vi "init UI.vi"(5 "Sub Panel":refnum<vi>, 6 "node ref":T9, 8 "Top VI":refnum<vi>, 9 "Enum in":refnum<vi>, 10 "Listbox":refnum<vi>, 11 "References in":T2) -> (0 "error out":errorcluster, 1 "Objects out":T1, 2 "Event Registration Refnum":refnum<event-registration>, 3 "References out":T2, 4 "Multi Column Listbox out":refnum<class "Multi Column Listbox.lvclass">)   [LabVIEW 2013, in "Scaling editor node.lvclass"]
uses:
  Scaling editor node.lvclass
  <vilib>/NI/Configuration Framework/Node/NodeRef.ctl
  <vilib>/NI/Configuration Framework/Node/NISE_CEF_Node.lvclass
  <vilib>/NI/DCAF Table API/Table Manager/references.ctl
  <vilib>/NI/Configuration Framework/Node/StopEvent.ctl
  <vilib>/NI/Configuration Framework/Node/RefreshUIEvent.ctl
  <vilib>/NI/Configuration Framework/Node/CacheState.ctl
  <vilib>/NI/Configuration Framework/Node/NodeChangeEvent.ctl
  <vilib>/NI/Tag Bus Data Framework/control module/editor node/channel action event.ctl
  <vilib>/NI/Tag Bus Data Framework/control module/editor node/dialog output action.ctl
  <vilib>/NI/Tag Bus Module Framework/channel/TBM channel.lvclass
  <vilib>/NI/Tag Bus/tag/tag descriptor.lvclass
  <vilib>/NI/AMC/Message Queue.ctl
  <vilib>/NI/AMC/Message.ctl
  <vilib>/NI/Tools/Keyed Array/KeyedArray.ctl
  <vilib>/NI/Configuration Framework/Node/UserEventRef.ctl
  <vilib>/NI/Configuration Framework/Controls/EventCluster.ctl
  <vilib>/NI/DCAF Table API/Table Manager/object ref.ctl
  <vilib>/NI/Tag Bus Data Framework/Configuration Editor/Classes/Engine Parent/Engine Parent Editor Node.lvclass
  <vilib>/NI/Tag Bus Data Framework/Configuration Editor/Classes/Module editor node/module editor node.lvclass
  <vilib>/NI/DCAF Table API/Listbox/Multi Column Listbox.lvclass
  <vilib>/NI/DCAF Table API/Listbox/Multi Column Listbox.lvclass/Multi Column Listbox.ctl
  <vilib>/NI/DCAF Table API/Table Manager/Table Manager.lvclass/Table Manager.ctl
  <vilib>/NI/DCAF Table API/Listbox/Write Listbox.vi
  <vilib>/NI/DCAF Table API/Table Manager/Write Top VI.vi
  <vilib>/NI/DCAF Table API/Table Manager/Table Manager.lvclass
  <vilib>/NI/Tag Bus Data Framework/control module/editor node/control module editor.lvclass
  <vilib>/NI/Tools/Keyed Array/Tools_KeyedArray.lvlib
  <vilib>/NI/AMC/AMC.lvlib
  <vilib>/NI/Configuration Framework/NISE_CEF_TreeControl.lvlib
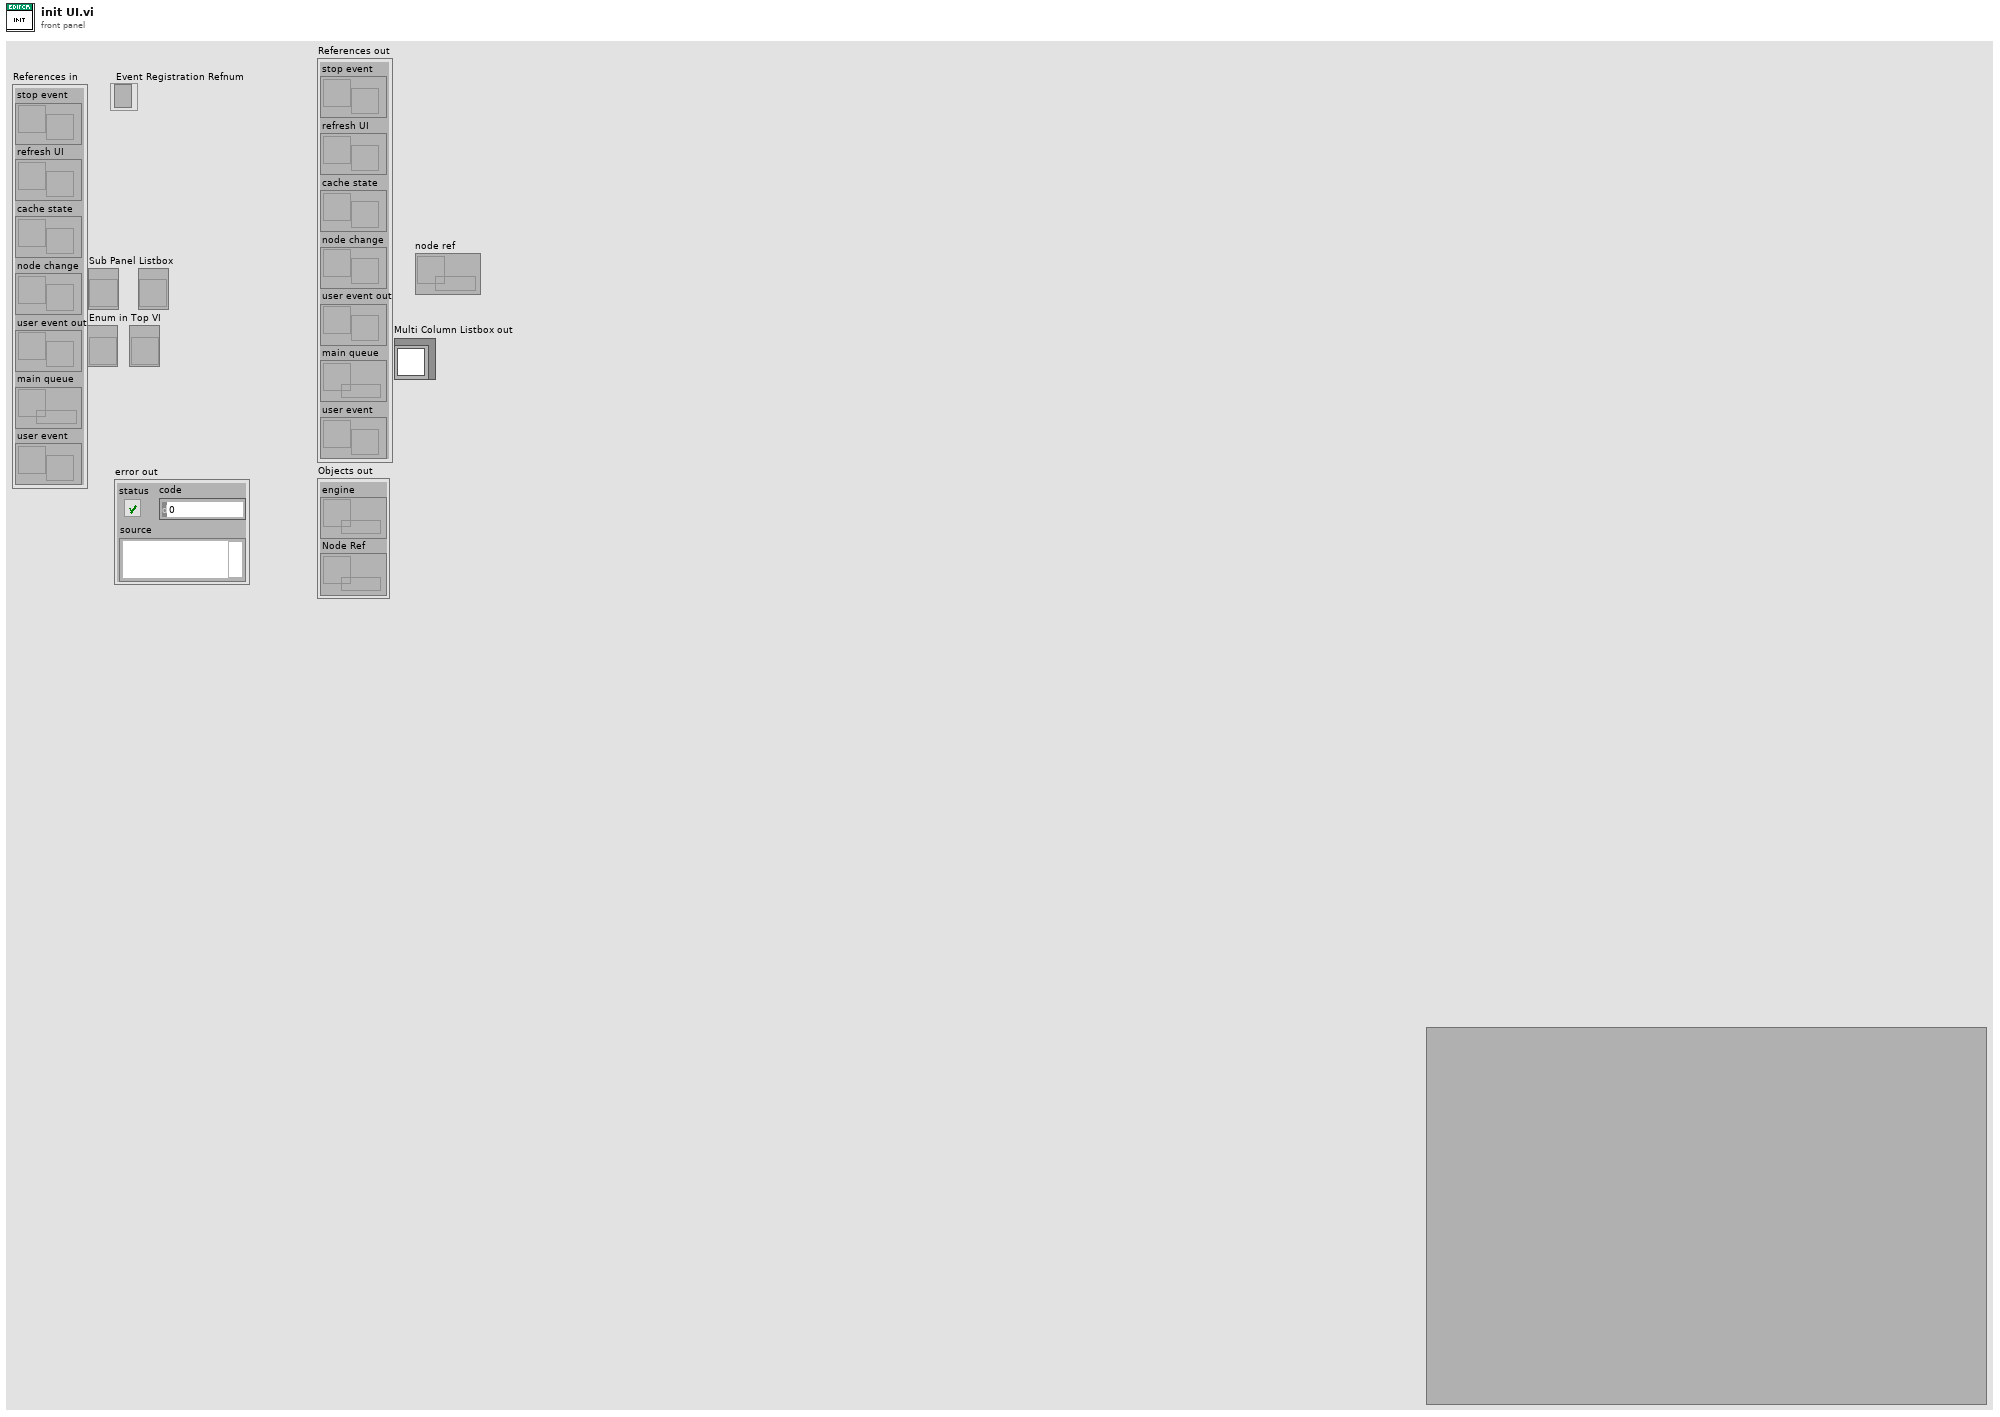
[diagram p1: front panel]
types:
  T1 = typedef "Table Manager.lvlib/Table Manager.lvclass/object ref.ctl" = cluster{"engine":refnum<data-value>, "Node Ref":refnum<data-value>}
  T2 = typedef "Table Manager.lvlib/Table Manager.lvclass/references.ctl" = cluster{"stop event":T3, "refresh UI":T4, "cache state":T5, "node change":T6, "user event out":refnum<user-event>, "main queue":T7, "user event":T8}
  T3 = typedef "NISE_CEF_Node.lvclass/StopEvent.ctl" = refnum<user-event>
  T4 = typedef "NISE_CEF_Node.lvclass/RefreshUIEvent.ctl" = refnum<user-event>
  T5 = typedef "NISE_CEF_Node.lvclass/CacheState.ctl" = refnum<user-event>
  T6 = typedef "NISE_CEF_Node.lvclass/NodeChangeEvent.ctl" = refnum<user-event>
  T7 = typedef "AMC.lvlib/Message Queue.ctl" = refnum<queue>
  T8 = typedef "NISE_CEF_Node.lvclass/UserEventRef.ctl" = refnum<user-event>
  T9 = typedef "NISE_CEF_Node.lvclass/NodeRef.ctl" = refnum<data-value>
  T10 = typedef "Table Manager.lvlib/Column.lvclass/Column Descriptor.ctl" = cluster{"name":string, "caption":string, "Column Type":T11, "Params":string, "AutoSizeMode":i32, "FillWeight":sgl, "MinWidth":u32, "tooltip":string, "Enum Reference":refnum<vi>, "Channel suffix":string, "Read Only":bool, "Call Back VI":T12, "DT Dependency":i32, "name dependency":i32, "data type":T13}
  T11 = typedef "Table Manager.lvlib/Column.lvclass/Column Type.ctl" = enum16{"String", "Mapping", "Channel Name", "Tag", "Enum", "Data Type", "Numeric"}
  T12 = typedef "Table Manager.lvlib/Table Manager.lvclass/Call Back Ref Type Def.ctl" = refnum<vi>
  T13 = typedef "tag bus.lvlib/tag descriptor.lvclass/Data Type.ctl" = enum16{"Double", "Single", "I64", "I32", "I16", "I8", "U64", "U32", "U16", "U8", "Boolean", "String", "Array of Double", "Array of Single", "Array of I64", "Array of I32", "Array of I16", "Array of I8", "Array of U64", "Array of U32", "Array of U16", "Array of U8", "Array of Boolean", "Array of String"}
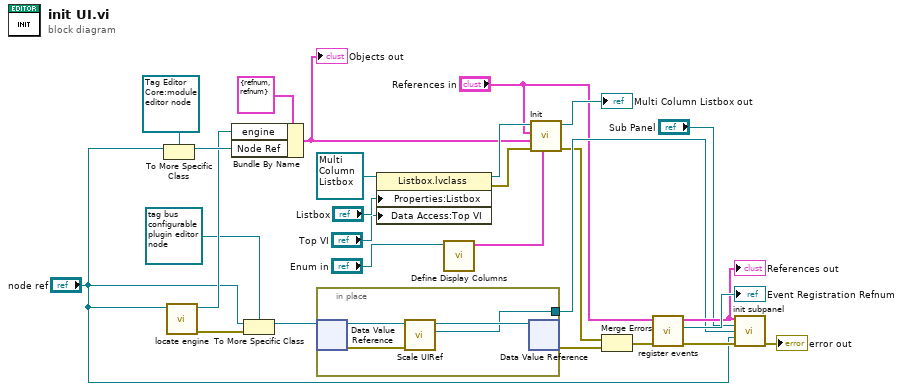
[diagram p0: block diagram]
diagram:
  n1 = To More Specific Class(target class=refnum<data-value> refnum ("data value reference"), reference="node ref") -> (specific class reference=w27:refnum<data-value>)  [unwired: 1 in, 1 out]
  n2 = call <vilib>:"locate engine.vi"("component"="node ref") -> ("error out"=w23:errorcluster, "engine"=w25:refnum<data-value>)  [unwired: 9 in]
  n3 = Bundle By Name(cluster=T1 {"engine"=refnum, "Node Ref"=refnum} ("object refs"), "engine"=w25, "Node Ref"=w27) -> (w2:T1)
  "Objects out" <- w2
  n4 = To More Specific Class(target class=refnum<data-value> refnum ("data value reference"), reference="node ref", error in=w23) -> (specific class reference=w19:refnum<data-value>)  [unwired: 1 out]
  n5 = in-place {
    in-place-border: [w28] -> w15
    n6 = in-place-dvr #1(w19) -> (w30:refnum<class "Scaling editor node.lvclass">, w31:errorcluster)
    n7 = call-dynamic "Scale UIRef.vi"("error in (no error)"=w31, "Scaling editor node in"=w30) -> ("VI refnum"=w28:refnum<vi>, "Scaling editor node out"=w29:refnum<class "Scaling editor node.lvclass">)  [unwired: 7 in, 1 out]
    n8 = in-place-dvr #1(w29) -> (w4:errorcluster)  [unwired: 1 out]
  }
  n9 = property class="Listbox.lvclass"(reference=refnum<class "Multi Column Listbox.lvclass"> refnum ("Multi Column Listbox in"), "Properties:Listbox"="Listbox", "Data Access:Top VI"="Top VI") -> (reference out=w11:refnum<class "Multi Column Listbox.lvclass">, error out=w10:errorcluster)  [unwired: 1 in]
  n10 = call "Define Display Columns.vi"("Enum in"="Enum in") -> ("Columns"=w13:T10[])  [unwired: 10 in]
  n11 = call-dynamic "Init.vi"("Column Definitions"=w13, "error in (no error)"=w10, "object refs"=w2, "References in"="References in", "Multi Column Listbox in"=w11) -> ("error out"=w5:errorcluster, "Multi Column Listbox out"=→"Multi Column Listbox out":refnum<class "Multi Column Listbox.lvclass">)  [unwired: 4 in, 1 out]
  n12 = Merge Errors(w5, w4) -> (w3:errorcluster)
  n13 = call "register events.vi"("error in (no error)"=w3, "References"="References in") -> ("error out"=w21:errorcluster, "Event Registration Refnum"=→"Event Registration Refnum":refnum<event-registration>, "References out"=w17:T2)  [unwired: 7 in]
  "References out" <- w17
  n14 = call "init subpanel.vi"("References in"=w17, "Sub Panel"="Sub Panel", "VI refnum"=w15, "node ref"="node ref", "error in (no error)"=w21) -> ("error IO"=→"error out":errorcluster)  [unwired: 10 in]
